vi "Dynamic Shared Variable and Alarm Example.vi"() -> ()   [LabVIEW 2018, in "Dynamic Shared Variables.lvlib"]
uses:
  Dynamic Shared Variables.lvlib
  URL Type Enum.ctl
  <vilib>/lvdsc/variables/internal/Configure Alarming (Shared Variable, Enable Alarming).vi
  <vilib>/lvdsc/variables/internal/Configure Alarming (Shared Variable, Numeric).vi
  <vilib>/lvdsc/alarm/Acknowledge Alarms By Variable Name.vi
  <vilib>/lvdsc/NI_DSC.lvlib
panel:
  in  "Tag Value":dbl(knob) scale=0.0..100.0
  out "URL":string
  out "string":string="\\\\.\\sv_alarm_example\\my_number"
  out "shared variable":refnum<k21>="\\\\.\\sv_alarm_example\\my_number"
  in  "numeric alarm settings":T1={"enable? (F)"=TRUE, "name"="HiHi", "alarm type"=enum."HI_HI", "level/change"=50.0, "deadband/time"=1.0, "priority"=1, "ack type"=enum."User", "area"="", "description"="", "log? (T)"=TRUE}
  out "process name out":string="sv_alarm_example"
  out "error out":errorcluster
  in  "stop":bool
  in  "Ack Button":bool
  in  "HiHi":dbl(knob) scale=0.0..100.0
  in  "HiHi Button":bool
  out "HiHi error out":errorcluster
  out "alarms":T2(array[cluster])=[{"alarm URL"="\\\\Nate-VM-LV2018\\sv_alarm_example\\my_number.Alarms.HiHi", "set time"=timestamp(3622821436.098553 s since 1904-01-01), "set user"="(Nobody)", "ack time"=timestamp(-9223372036854775808 s since 1904-01-01), "ack user"="", "clear time"=timestamp(-9223372036854775808 s since 1904-01-01), "clear user"="", "setpoint"=50.0, "value"=97.88238901880113, "priority"=1, "alarm area"="", "alarm description"="", "ack comment"="", "event?"=FALSE, "Refnum"=216172782113783811}] {"value" format="%.2f"; "setpoint" format="%.2f"; "clear time" format="%<%X\n%x>T"; "ack time" format="%<%X\n%x>T"; "set time" format="%<%X\n%x>T"}
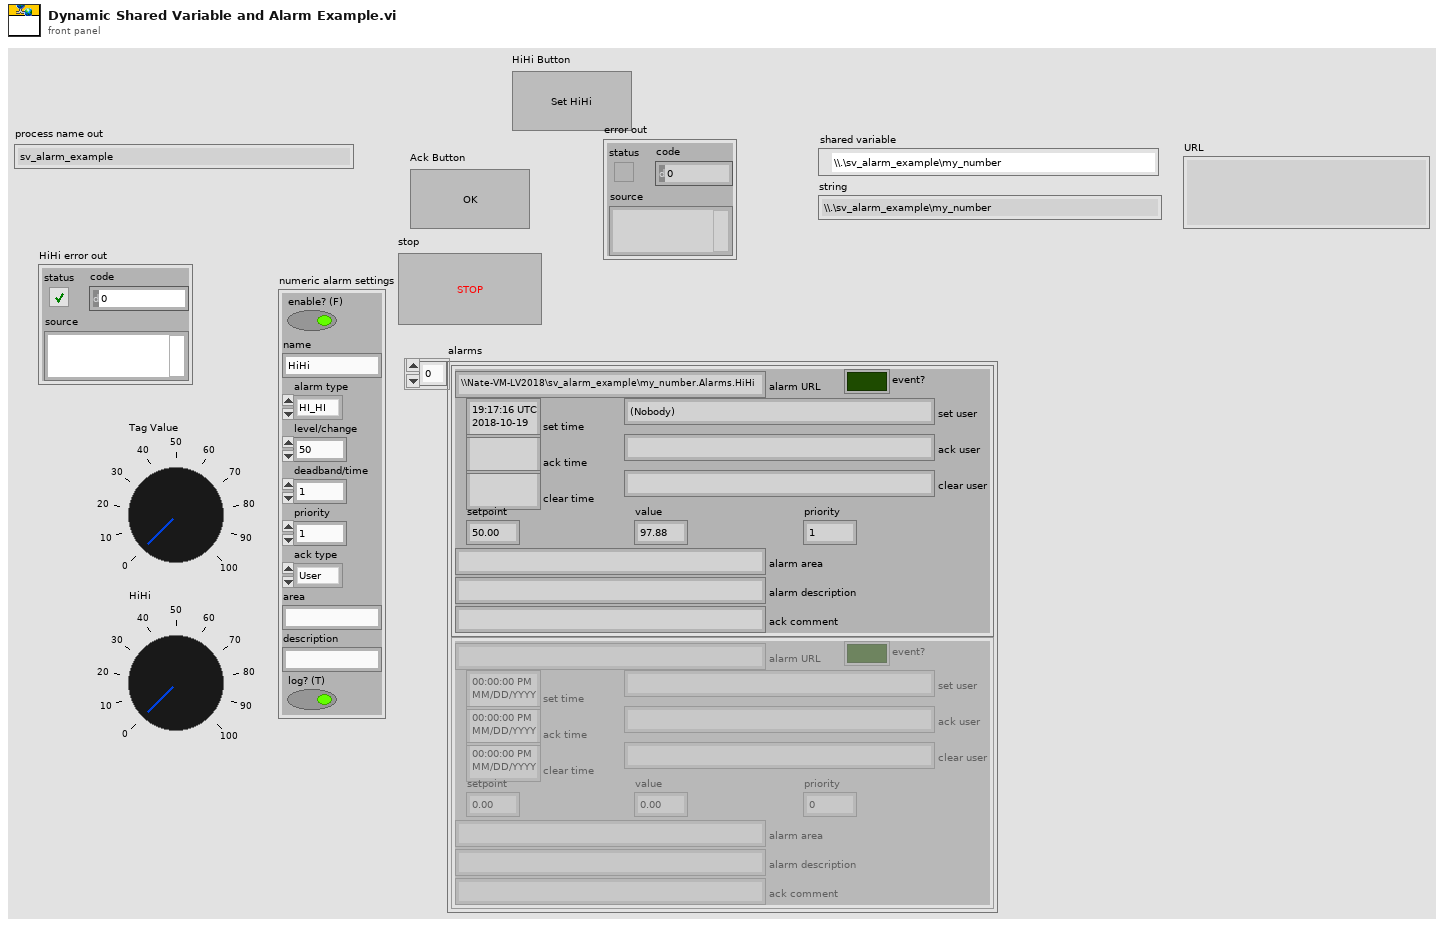
[diagram p1: front panel]
types:
  T1 = cluster{"enable? (F)":bool, "name":string, "alarm type":enum16{"HI_HI", "HI", "LO", "LO_LO"}, "level/change":dbl, "deadband/time":dbl, "priority":u32, "ack type":enum16{"Auto", "User", "None", "Each Occurrence"}, "area":string, "description":string, "log? (T)":bool}
  T2 = cluster{"alarm URL":string, "set time":timestamp, "set user":string, "ack time":timestamp, "ack user":string, "clear time":timestamp, "clear user":string, "setpoint":dbl, "value":dbl, "priority":u32, "alarm area":string, "alarm description":string, "ack comment":string, "event?":bool, "Refnum":u64}[]
  T3 = typedef "Dynamic Shared Variables.lvlib/URL Type Enum.ctl" = enum16{"Tag", "HiHi", "Hi", "Lo", "LoLo"}
  T4 = cluster{"use binding? (F)":bool, "URL":string, "access type":enum32{"Read only", "Write only", "Read/write"}, "buffer size":u32, "use buffering? (F)":bool, "single writer? (F)":bool}
  T5 = enum32{"u32BitField", "bool", "double", "string", "int8", "uint8", "int16", "uint16", "int32", "uint32", "int64", "uint64", "single", "double waveform", "int16 waveform", "array of boolean", "array of int8", "array of uint8", "array of int16", "array of uint16", "array of int32", "array of uint32", "array of int64", "array of uint64", "array of single", "array of double", "array of double waveform", "array of int16 waveform", "array of string", "variant", "timestamp", "fixed point", "custom"}
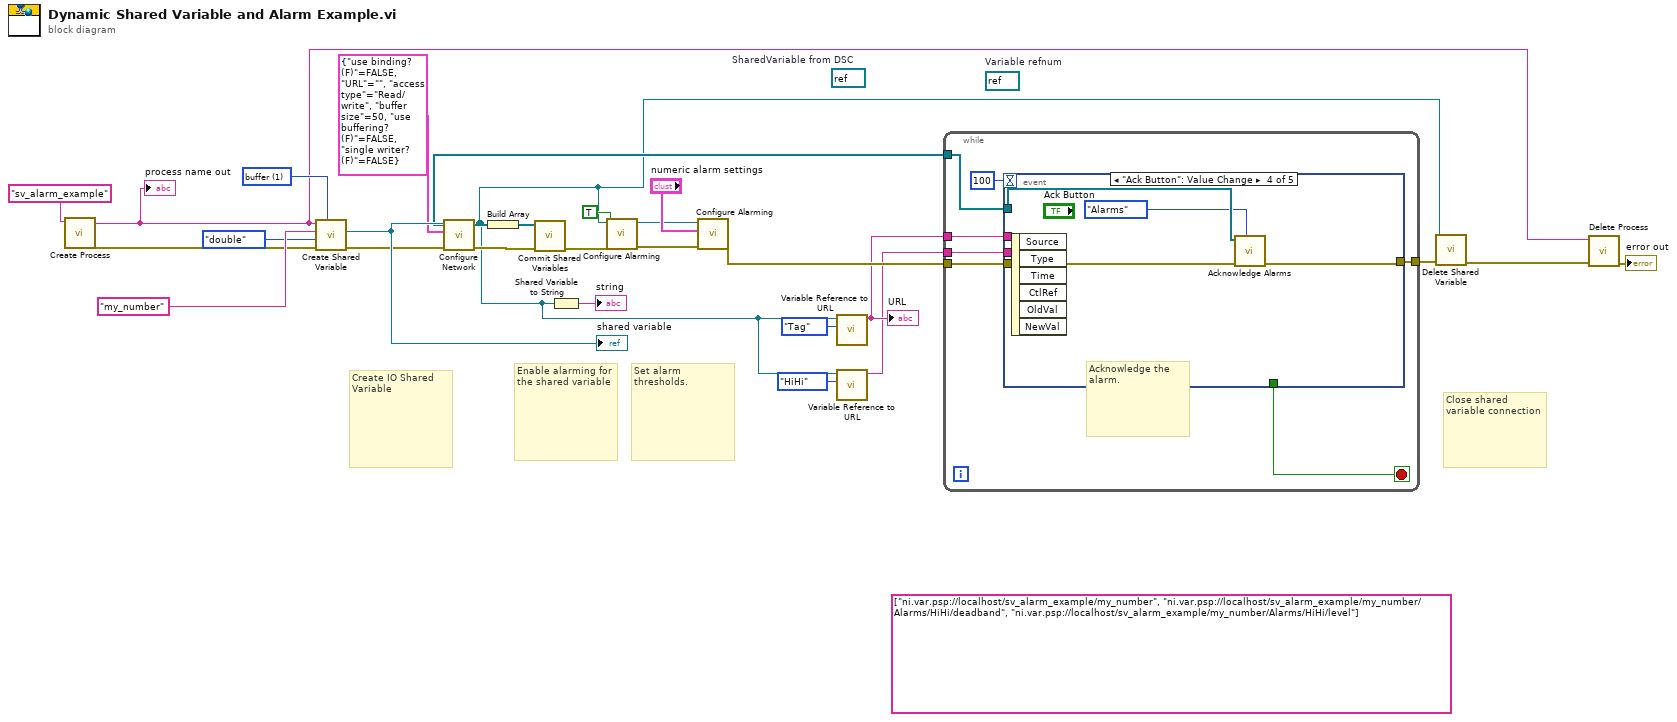
[diagram p0: block diagram]
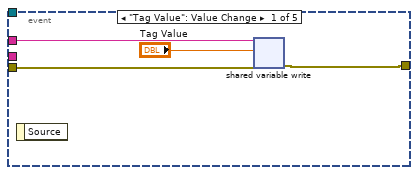
[diagram p2: hidden frame]
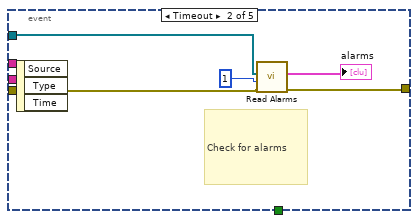
[diagram p3: hidden frame]
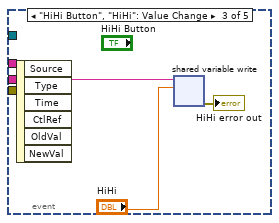
[diagram p4: hidden frame]
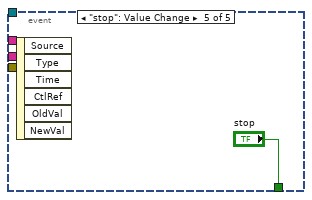
[diagram p5: hidden frame]
diagram:
  (unwired) refnum<k21> refnum  # SharedVariable from DSC
  (unwired) refnum<k21> refnum  # Variable refnum
  (unwired) string[] ["ni.var.psp://localhost/sv_alarm_example/my_number", "ni.var.psp://localhost/sv_alarm_example/my_number/Alarms/HiHi/deadband", "ni.var.psp://localhost/sv_alarm_example/my_number/Alarms/HiHi/level"] ("URL 2")
  w26 = u16 1 items=["commit", "buffer"] ("set mode")
  # "Close shared variable connection"
  # "Create IO Shared Variable"
  # "Set alarm thresholds."
  # "Enable alarming for the shared variable"
  n1 = call "Create Process.vi"("process name"="sv_alarm_example") -> ("error out"=w22:errorcluster, "process name out"=w15:string)  [unwired: 9 in]
  "process name out" <- w15
  n2 = call <vilib>:"Create Shared Variable.vi"("set mode"=w26, "error in (no error)"=w22, "data type"=T5."double", "shared variable name"="my_number", "process name"=w15) -> ("error out"=w20:errorcluster, "shared variable"=w21:refnum<k21>)  [unwired: 4 in, 1 out]
  "shared variable" <- w21
  n3 = call <vilib>:"Configure Network.vi"("error in (no error)"=w20, "network settings"=T4 {"use binding? (F)"=FALSE, "URL"="", "access type"=enum."Read/write", "buffer size"=50, "use buffering? (F)"=FALSE, "single writer? (F)"=FALSE}, "variable reference in"=w21) -> ("error out"=w18:errorcluster, "variable reference out"=w2:refnum<k21>)  [unwired: 7 in]
  n4 = Build Array(w2) -> (w13:refnum<k21>[])
  n5 = call <vilib>:"Commit Shared Variables.vi"("error in (no error)"=w18, "shared variables"=w13) -> ("error out"=w11:errorcluster)  [unwired: 8 in, 1 out]
  n6 = Shared Variable to String(1:w2) -> (0:→"string":string)
  n7 = call-poly <vilib>:"Configure Alarming.vi"("error in (no error)"=w11, "enable? (F)"=TRUE, "variable reference in"=w2) -> ("error out"=w9:errorcluster, "variable reference out"=w10:refnum<k21>)  [unwired: 7 in]
  n8 = call-poly <vilib>:"Configure Alarming.vi"("error in (no error)"=w9, "numeric alarm settings"="numeric alarm settings", "variable reference in"=w10) -> ("error out"=w8:errorcluster)  [unwired: 7 in, 1 out]
  n9 = call "Variable Reference to URL.vi"("URL type"=URL_Type_Enum."Tag", "variable reference"=w2) -> ("URL"=w5:string)  [unwired: 8 in, 1 out]
  "URL" <- w5
  n10 = call "Variable Reference to URL.vi"("URL type"=URL_Type_Enum."HiHi", "variable reference"=w2) -> ("URL"=w1:string)  [unwired: 8 in, 1 out]
  n11 = while {
    tunnel: w8 -> [w33]
    tunnel: w5 -> [w31]
    tunnel: [w30] -> w4
    tunnel: w13 -> [w29]
    tunnel: w1 -> [w28]
    stop <- w32 stop-if-true
    n12 = event shown="[3] \"Ack Button\": Value Change" {
      selector: _ -> [_ _ _ _ _]
      dyn-events: _ -> [_ _ _ _ _]
      timeout: 100 -> [_ _ _ _ _]
      tunnel: w31 -> [w37 _ _ _ _]
      tunnel: w33 -> [w36 w39 _ w49 _]
      tunnel: [_ _ _ _ "stop"] -> w32
      tunnel: [w34 w42 _ w48 _] -> w30
      tunnel: w29 -> [_ w41 _ w47 _]
      tunnel: w28 -> [_ _ w43 _ _]
      event "Tag Value": Value Change {
        n13 = event-data() -> ()  [unwired: 1 in, 1 out]
        n14 = shared-variable-write(w37, w36, "Tag Value") -> (w34:errorcluster)  [unwired: 1 out]
      }
      event Timeout {
        # "Check for alarms"
        n15 = event-data() -> ()  [unwired: 1 in, 3 out]
        n16 = call <vilib>:"Read Alarms.vi"("error in (no error)"=w39, "timeout (s)"=1, "shared variables"=w41) -> ("error out"=w42:errorcluster, "alarms"=→"alarms":T2)  [unwired: 7 in]
      }
      event "HiHi Button", "HiHi": Value Change {
        n17 = event-data() -> ()  [unwired: 1 in, 6 out]
        n18 = shared-variable-write(w43, "HiHi") -> (→"HiHi error out":errorcluster)  [unwired: 1 in, 1 out]
      }
      event "Ack Button": Value Change {
        # "Acknowledge the alarm."
        n19 = event-data() -> ()  [unwired: 1 in, 6 out]
        n20 = call-poly <vilib>:"Acknowledge Alarms.vi"("acknowledge type"=enum16{"Alarms", "Events", "Alarms & Events"}."Alarms", "error in (no error)"=w49, "shared variables"=w47) -> ("error out"=w48:errorcluster)  [unwired: 8 in]
      }
      event "stop": Value Change {
        n21 = event-data() -> ()  [unwired: 1 in, 6 out]
      }
    }
  }
  n22 = call <vilib>:"Delete Shared Variable.vi"("error in (no error)"=w4, "shared variable"=w2) -> ("error out"=w16:errorcluster)  [unwired: 9 in]
  n23 = call <vilib>:"Delete Process.vi"("error in (no error)"=w16, "process name"=w15) -> ("error out"=→"error out":errorcluster)  [unwired: 9 in]
